vi "uPython_Close.vi"(8 "error in":errorcluster, 11 "VISA  in":refnum<visa-resource-name>) -> (0 "error out":errorcluster, 3 "VISA  out":refnum<visa-resource-name>)   [LabVIEW 2016]
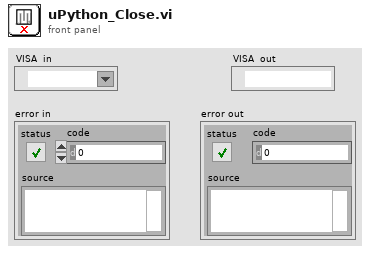
[diagram p1: front panel]
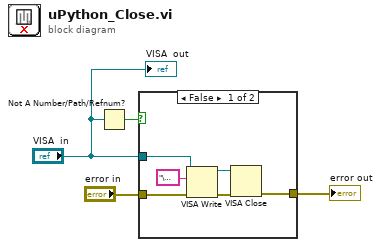
[diagram p0: block diagram]
diagram:
  n1 = Not A Number/Path/Refnum?(number/path/refnum="VISA  in") -> (NaN/Path/Refnum?=w1:bool)
  n2 = case shown="False" w1 {
    tunnel: [w10 w11] -> w4
    tunnel: "error in" -> [w9 w11]
    tunnel: "VISA  in" -> [w8 _]
    frame False {
      n3 = VISA Write(VISA resource name=w8, write buffer="\u0003", error in (no error)=w9) -> (VISA resource name out=w7:refnum<visa-resource-name>, error out=w6:errorcluster)  [unwired: 1 out]
      n4 = VISA Close(VISA resource name=w7, error in (no error)=w6) -> (error out=w10:errorcluster)
    }
    frame True {
    }
  }
  "error out" <- w4
  "VISA  out" <- "VISA  in"
